vi "Teardown.vi"(11 "Dev Actor in":refnum<class "Dev Actor.lvclass">) -> (3 "Dev Actor out":refnum<class "Dev Actor.lvclass">)   [LabVIEW 2021, in "Dev Actor.lvlib" / "Dev Actor.lvclass"]
uses:
  Dev Actor.lvclass
  Dev Actor.lvclass/Dev Actor.ctl
  <vilib>/jettl/jettl/Actor/Actor/Actor.lvclass
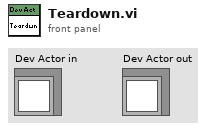
[diagram p1: front panel]
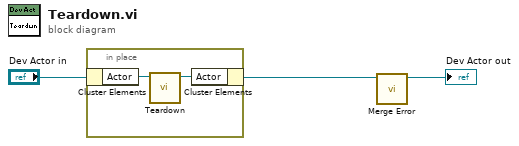
[diagram p0: block diagram]
diagram:
  n1 = in-place {
    n2 = in-place-cluster #1("Dev Actor in") -> ("Actor"=w5:refnum<class "Actor.lvclass">)
    n3 = call-dynamic "Teardown.vi"("Teardown in"=w5) -> ("Teardown out"=w4:refnum<class "Actor.lvclass">)  [unwired: 10 in]
    n4 = in-place-cluster #1("Actor"=w4) -> (w1:refnum<class "Dev Actor.lvclass">)
  }
  n5 = call-dynamic "Merge Error.vi"("Dev Actor in"=w1) -> ("Dev Actor out"=→"Dev Actor out":refnum<class "Dev Actor.lvclass">)  [unwired: 10 in]
